vi "Synchonize Relay States.vi"(8 "error in (no error)":errorcluster, 11 "SLSC Switch in":refnum<class "SLSC Switch.lvclass">) -> (0 "error out":errorcluster, 3 "SLSC Switch out":refnum<class "SLSC Switch.lvclass">)   [LabVIEW 2015, in "SLSC Switch.lvclass"]
uses:
  SLSC Switch.lvclass
  SLSC Switch.lvclass/SLSC Switch.ctl
  Relay Interface/RelayInterface.lvclass
  slscsl/slscsl.lvclass
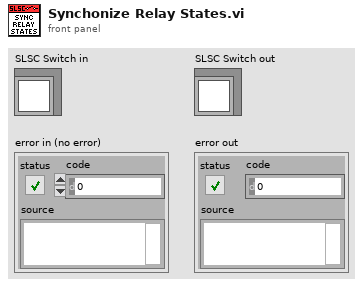
[diagram p1: front panel]
types:
  T1 = typedef "slscsl.lvclass/RelayPosition.ctl" = i32
  T2 = typedef "slscsl.lvclass/RelayAction.ctl" = u32
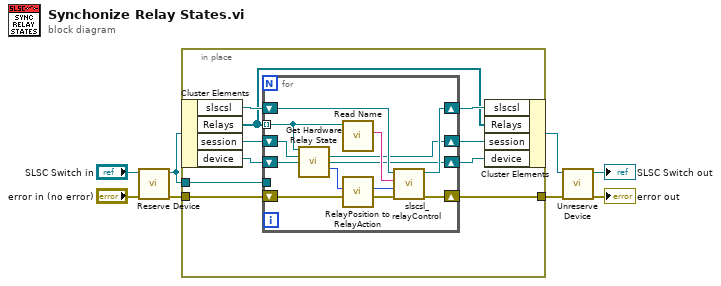
[diagram p0: block diagram]
diagram:
  n1 = call "Reserve Device.vi"("error in (no error)"="error in (no error)", "SLSC Switch in"="SLSC Switch in") -> ("error out"=w3:errorcluster, "SLSC Switch out"=w4:refnum<class "SLSC Switch.lvclass">)  [unwired: 8 in]
  n2 = in-place {
    in-place-border: [w18] -> w6
    in-place-border: w4 -> [w17]
    in-place-border: w3 -> [w16]
    n3 = in-place-cluster #1(w4) -> ("slscsl"=w15:refnum<class "slscsl.lvclass">, "Relays"=w13:refnum<class "RelayInterface.lvclass">[], "session"=w11:refnum<k21>, "device"=w10:refnum<k21>)
    n4 = for {
      tunnel: w13 -> [w24] mode=indexing
      tunnel: w17 -> [_]
      shift-right: [w28] -> w14
      shift-left: w15 -> [w29]
      shift-right: [w27] -> w18
      shift-left: w16 -> [w30]
      shift-right: [w20] -> w9
      shift-left: w10 -> [w22]
      shift-right: [w21] -> w12
      shift-left: w11 -> [w23]
      n5 = call-dynamic "Get Hardware Relay State.vi"("RelayInterface in"=w24, "session in"=w23, "device in"=w22) -> ("session out"=w21:refnum<k21>, "device out"=w20:refnum<k21>, "RelayPosition"=w19:T1)  [unwired: 8 in, 2 out]
      n6 = call-dynamic "Read Name.vi"("RelayInterface in"=w24) -> ("Name"=w25:string)  [unwired: 9 in, 1 out]
      n7 = call "RelayPosition to RelayAction.vi"("position"=w19) -> ("action"=w26:T2)  [unwired: 10 in]
      n8 = call "slscsl_relayControl.vi"("error in (no error)"=w30, "RelayAction"=w26, "relayNames"=w25, "slscsl in"=w29) -> ("error out"=w27:errorcluster, "slscsl out"=w28:refnum<class "slscsl.lvclass">)  [unwired: 5 in, 1 out]
    }
    n9 = in-place-cluster #1("slscsl"=w14, "Relays"=w13, "session"=w12, "device"=w9) -> (w5:refnum<class "SLSC Switch.lvclass">)
  }
  n10 = call "Unreserve Device.vi"("error in (no error)"=w6, "SLSC Switch in"=w5) -> ("error out"=→"error out":errorcluster, "SLSC Switch out"=→"SLSC Switch out":refnum<class "SLSC Switch.lvclass">)  [unwired: 8 in]
